vi "SV Measure Delay.vi"   [LabVIEW 2017, in "SoundVib_Calibration.lvlib"]
doc: "Use this VI to measure the propagation delay of a response signal. Use this VI when performing stimulus-response measurements to polarity normalize and time align the response signals prior to precision block processing. Use the equal polarity instance when the delayed signal exhibits equal polarity and simple time delay."
uses:
  <vilib>/addons/Sound and Vibration/svt_Calibration/SoundVib_Calibration.lvlib
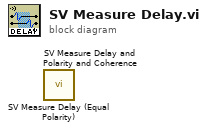
[diagram p0: block diagram]
diagram:
  n1 = call <vilib>:"SV Measure Delay (Equal Polarity).vi"() -> ()  [unwired: 13 in, 3 out]
  n2 = call <vilib>:"SV Measure Delay and Polarity and Coherence.vi"() -> ()  [unwired: 11 in, 5 out]
